vi "set data.vi"() -> ()   [LabVIEW 2018]
panel:
  out "错误代码":u16 format="%04x"
  out "写入状态":bool
  in  "数组":i16[](array[numeric])=[4321]
  in  "软元件":string="D0"
  in  "本地端口":u16=65502
  in  "目的端口":u16=65502
  in  "目的IP地址":string="192.168.3.250"
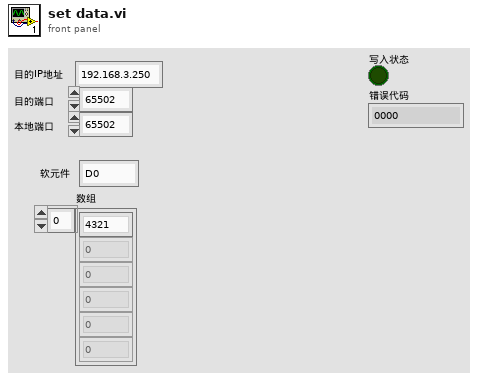
[diagram p1: front panel]
types:
  T1 = cluster{"目的端口":u16, "网络地址":u32, "连接ID":refnum<k16>}
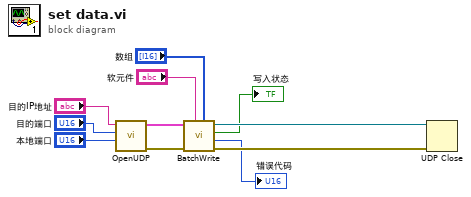
[diagram p0: block diagram]
diagram:
  n1 = call "OpenUDP.vi"("本地端口"="本地端口", "目的端口"="目的端口", "目的IP地址"="目的IP地址") -> ("错误输出"=w11:errorcluster, "连接输出"=w1:T1)  [unwired: 7 in]
  n2 = call "BatchWrite.vi"("输入数组"="数组", "软元件"="软元件", "错误输入"=w11, "连接输入"=w1) -> ("错误输出"=w9:errorcluster, "错误代码"=→"错误代码":u16, "写入状态"=→"写入状态":bool, "连接ID OUT"=w10:refnum<k16>)  [unwired: 4 in]
  n3 = UDP Close(connection ID=w10, 8:w9) -> ()  [unwired: 2 out]
